vi "AE Cam# 2.vi"(7 "update":bool, 11 "Cam#":i32) -> (3 "Cam# out":i32)   [LabVIEW 2025]
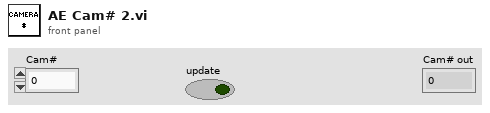
[diagram p1: front panel]
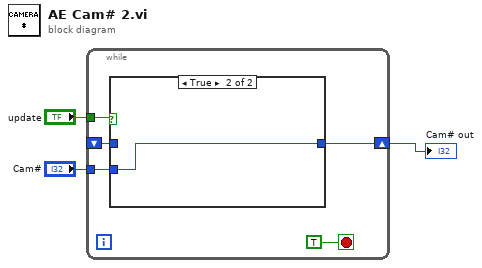
[diagram p0: block diagram]
diagram:
  n1 = while {
    shift-right: [w6] -> w1
    shift-left: _ -> [w5]
    tunnel: "Cam#" -> [w7]
    tunnel: "update" -> [w4]
    stop <- TRUE stop-if-true
    n2 = case shown="True" w4 {
      tunnel: w7 -> [_ w10]
      tunnel: [w9 w10] -> w6
      tunnel: w5 -> [w9 _]
      frame False {
      }
      frame True {
      }
    }
  }
  "Cam# out" <- w1
